vi "Create Transfer.vi"(8 "error in (no error)":errorcluster, 10 "Transfer Configuration":T1, 11 "Transfer Configuration in":refnum<class "Transfer Configuration.lvclass">) -> (0 "error out":errorcluster, 3 "Transfer Configuration out":refnum<class "Transfer Configuration.lvclass">)   [LabVIEW 2017, in "Data Sharing Framework Engine.lvlib" / "Transfer Configuration.lvclass"]
uses:
  Transfer Configuration.lvclass
  old/dsf core/Source/DSF Configuration API/1.0.0/Public/Controls/DSF Engine Transfer Configuration.ctl
  old/dsf core/Source/DSF Configuration API/1.0.0/Public/Controls/DSF Byte Order.ctl
  old/dsf core/Source/DSF Configuration API/1.0.0/Public/Controls/DSF Engine Channel Configuration.ctl
  old/dsf core/Source/DSF Configuration API/1.0.0/Public/Controls/DSF Data Type.ctl
  old/dsf core/Source/DSF Configuration API/1.0.0/Public/Controls/DSF Settings Info.ctl
  old/dsf core/Source/DSF Configuration API/1.0.0/Public/Controls/DSF Direction.ctl
  old/dsf core/Source/DSF Configuration API/1.0.0/DSF Configuration API.lvlib
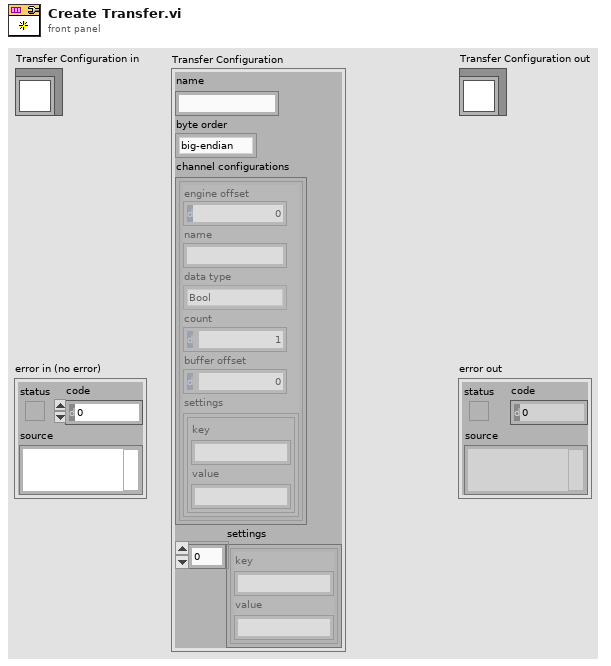
[diagram p1: front panel]
types:
  T1 = typedef "DSF Configuration API.lvlib/DSF Engine Transfer Configuration.ctl" = cluster{"name":string, "byte order":T2, "channel configurations":T3[], "settings":T5}
  T2 = typedef "DSF Configuration API.lvlib/DSF Byte Order.ctl" = enum8{"big-endian", "little-endian"}
  T3 = typedef "DSF Configuration API.lvlib/DSF Engine Channel Configuration.ctl" = cluster{"engine offset":u64, "name":string, "data type":T4, "count":u64, "buffer offset":u64, "settings":T5}
  T4 = typedef "DSF Configuration API.lvlib/DSF Data Type.ctl" = enum8{"Bool", "SGL", "DBL", "I8", "I16", "I32", "I64", "U8", "U16", "U32", "U64"}
  T5 = typedef "DSF Configuration API.lvlib/DSF Settings Info.ctl" = cluster{"key":string, "value":string}[]
  T6 = typedef "DSF Configuration API.lvlib/DSF Direction.ctl" = enum8{"Tx", "Rx"}
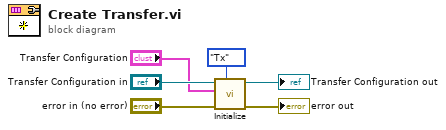
[diagram p0: block diagram]
diagram:
  n1 = call-dynamic "Initialize.vi"("direction"=DSF_Direction."Tx", "error in (no error)"="error in (no error)", "Transfer Configuration cluster"="Transfer Configuration", "Transfer Configuration in"="Transfer Configuration in") -> ("error out"=→"error out":errorcluster, "Transfer Configuration out"=→"Transfer Configuration out":refnum<class "Transfer Configuration.lvclass">)  [unwired: 6 in]
